vi "CSDB_Config.get AttributeID.vi"(3 "AttributeName":string, 5 "error in (no error)":errorcluster) -> (17 "AttributeID":string, 19 "error out":errorcluster)   [LabVIEW 2014, in "CSDB_Config.lvlib"]
doc: "Gets the ID of an attribute element."
uses:
  CSDB_Config.lvlib
  <vilib>/addons/database/_DB Variant To Data/Database Variant To Data.xnode
  <vilib>/addons/database/NI_Database_API.lvlib
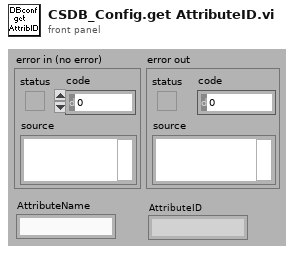
[diagram p1: front panel]
types:
  T1 = typedef "NI_Database_API.lvlib/Conn ObjectReference.ctl" = refnum<k1>
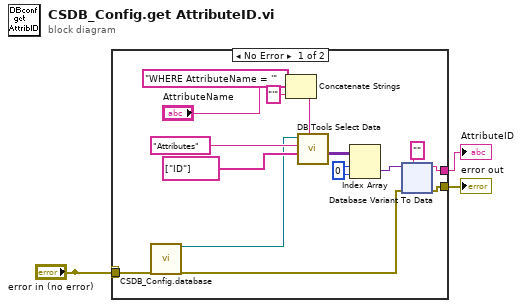
[diagram p0: block diagram]
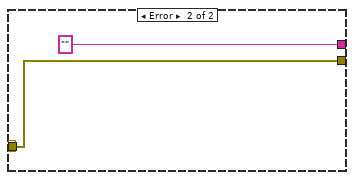
[diagram p2: hidden frame]
diagram:
  n1 = case shown="No Error" "error in (no error)" {
    tunnel: "error in (no error)" -> [w18 w52]
    tunnel: [w6 w52] -> w3
    tunnel: [w5 ""] -> w2
    frame No Error {
      w10 = 0 ("index (row)")
      n2 = call "CSDB_Config.database.vi"("error in (no error)"=w18) -> ("connectionRef out"=w4:T1, "error out"=w7:errorcluster)  [unwired: 17 in]
      n3 = Concatenate Strings("WHERE AttributeName = '" ("optional clause"), "AttributeName", "'" ("string")) -> (w12:string)
      n4 = call <vilib>:"DB Tools Select Data.vi"("condition"=w12, "columns"=string[] ["ID"], "table"="Attributes", "connection reference"=w4) -> ("data"=w11:variant[][])  [unwired: 2 in, 2 out]
      n5 = Index Array(array=w11, index (row)=w10, index (col)=w10) -> (element=w9:variant)
      n6 = xnode "Database Variant To Data"("database variant"=w9, "error in (no error)"=w7, "type"="") -> ("data"=w5:string, "error out"=w6:errorcluster)
    }
    frame Error {
    }
  }
  "error out" <- w3
  "AttributeID" <- w2
